vi "AbortServo.vi"(8 "error in":errorcluster, 11 "powerServoSession":u32) -> (0 "error out":errorcluster, 3 "powerServoSessionOut":u32)   [LabVIEW 2016, in "Power Servo.lvlib"]
uses:
  Power Servo.lvlib
  <userlib>/_NI Power Servoing IP/HostRdl/NI Power Servoing IP New (Host).lvlib
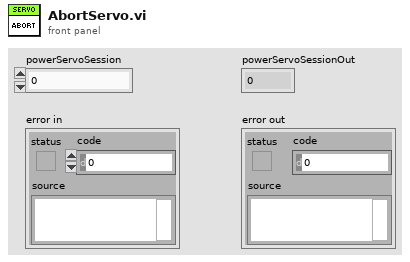
[diagram p1: front panel]
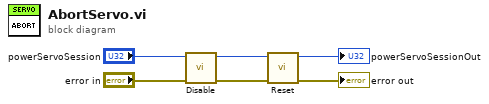
[diagram p0: block diagram]
diagram:
  n1 = call <userlib>:"Disable.vi"("error in"="error in", "SessionHandleIn"="powerServoSession") -> ("error out"=w3:errorcluster, "SessionHandleOut"=w4:u32)  [unwired: 8 in]
  n2 = call <userlib>:"Reset.vi"("error in"=w3, "SessionHandleIn"=w4) -> ("error out"=→"error out":errorcluster, "SessionHandleOut"=→"powerServoSessionOut":u32)  [unwired: 8 in]
